vi "CalcLift.vi"(5 "Teleop Local Data In":T1 {"Vision"."Theta_Y" format="%.1f"; "Vision"."Theta_X" format="%.1f"; "Potentio" format="%.1f"; "Drive_Enc_R" format="%.1f"; "Drive_Enc_L" format="%.1f"; "Gyro_Angle" format="%.1f"; "Encoder_Lift" format="%.1f"; "Motor_Lift" format="%.3f"; "Motor_Intake" format="%.3f"; "Drive_Twist" format="%.3f"; "Drive_Forward" format="%.3f"}, 9 "error in":errorcluster) -> (6 "Teleop Local Data Out":T1 {"Vision"."Theta_Y" format="%.1f"; "Vision"."Theta_X" format="%.1f"; "Potentio" format="%.1f"; "Drive_Enc_R" format="%.1f"; "Drive_Enc_L" format="%.1f"; "Gyro_Angle" format="%.1f"; "Encoder_Lift" format="%.1f"; "Motor_Lift" format="%.3f"; "Motor_Intake" format="%.3f"; "Drive_Twist" format="%.3f"; "Drive_Forward" format="%.3f"}, 10 "error out":errorcluster)   [LabVIEW 2018]
uses:
  Typedefs/typedef_cluster_TeleOp_Local_Data.ctl
  Typedefs/typedef_cluster_Joystick.ctl
  Typedefs/typedef_cluster_Vision.ctl
  Typedefs/typedef_enum_refnums.ctl
  <vilib>/Rock Robotics/WPI/ThirdParty/Phoenix-LabVIEW/Motor Controller/Get/CTRE_Phoenix_MotorController_GetQuadratureData.vi
  <vilib>/Rock Robotics/WPI/ThirdParty/Phoenix-LabVIEW/Motor Controller/Get/CTRE_Phoenix_MotorController_GetLimitSwitchStates.vi
panel:
  in  "K Down":dbl=8.0
  in  "K":dbl=5.0
  in  "lower limit":dbl
  in  "upper limit":dbl=2700.0
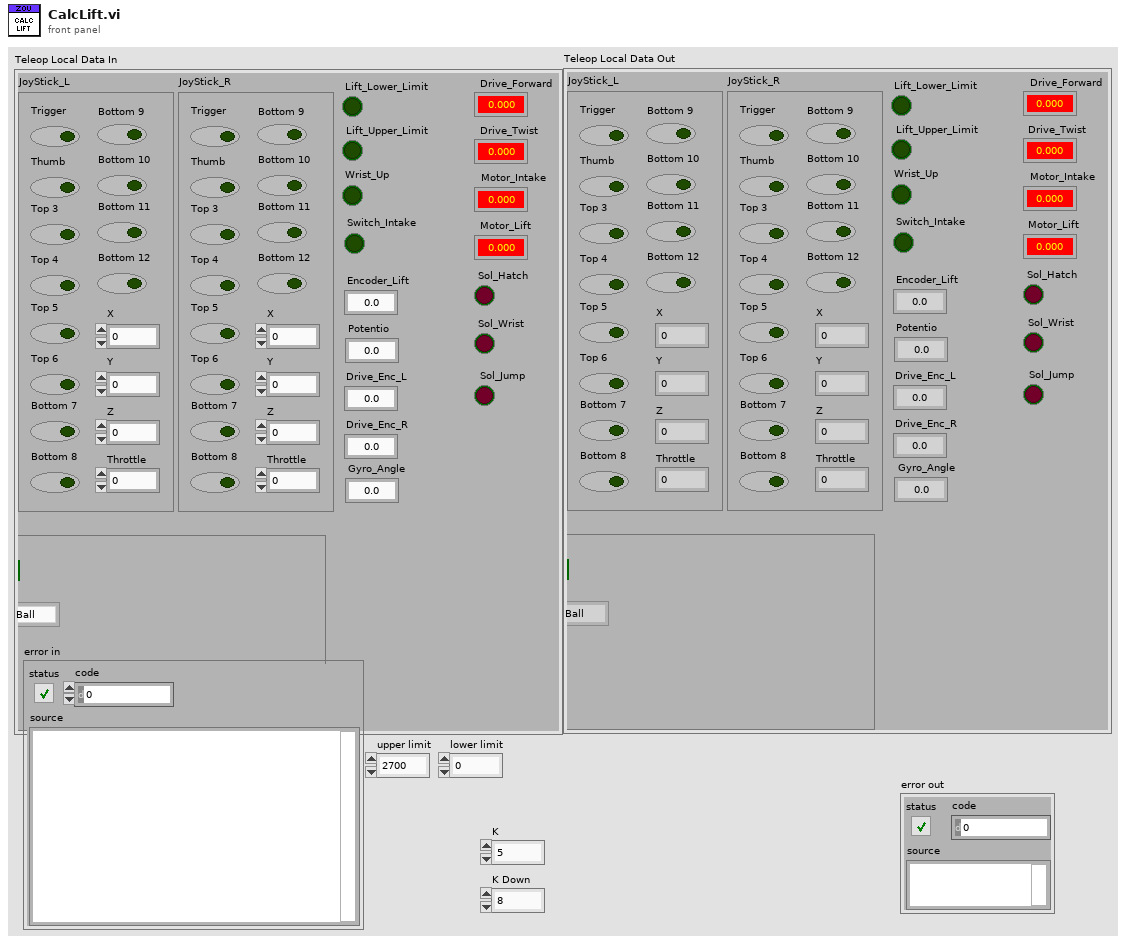
[diagram p1: front panel]
types:
  T1 = typedef "typedef_cluster_TeleOp_Local_Data.ctl" = cluster{"Lift_Lower_Limit":bool, "Wrist_Up":bool, "Switch_Intake":bool, "Encoder_Lift":dbl, "Sol_Wrist":bool, "Motor_Intake":dbl, "Motor_Lift":dbl, "Drive_Forward":dbl, "Drive_Twist":dbl, "Sol_Hatch":bool, "Gyro_Angle":dbl, "Drive_Enc_L":dbl, "Drive_Enc_R":dbl, "JoyStick_L":T2, "JoyStick_R":T2, "Potentio":dbl, "Vision":T3, "Lift_Upper_Limit":bool, "Sol_Jump":bool}
  T2 = typedef "typedef_cluster_Joystick.ctl" = cluster{"X":dbl, "Y":dbl, "Z":dbl, "Throttle":dbl, "Trigger":bool, "Thumb":bool, "Top 3":bool, "Top 4":bool, "Top 5":bool, "Top 6":bool, "Bottom 7":bool, "Bottom 8":bool, "Bottom 9":bool, "Bottom 10":bool, "Bottom 11":bool, "Bottom 12":bool}
  T3 = typedef "typedef_cluster_Vision.ctl" = cluster{"Theta_X":dbl, "Theta_Y":dbl, "Has_Target":bool, "Seek_Ball":bool, "Pipeline":enum16{"Ball", "Dual_Target", "Single_Target"}}
  T4 = typedef "typedef_enum_refnums.ctl" = enum16{"Joy_L", "Joy_R", "Drive_Motors", "Intake_Motor", "Wrist_Solenoid", "Hatch_Solenoid", "Compressor", "Lift_Motor", "Lift_Motor_2", "Gyro", "Drive_Enc_L", "Drive_Enc_R", "Lift_Lower_Limit", "Lift_Upper_Limit", "Ball_Switch", "Jump_Solenoid"}
  T5 = typedef "WPI_MotorControlDeviceRef.ctl" = cluster{"DeviceStatus":errorcluster, "Type":T6, "PWM":cluster{"PWM Channel":T7, "DeadBand":T8}, "CAN":cluster{"Device Number":u8, "SetOutput VI Ref":variant, "GetOutput VI Ref":variant, "Enable VI Ref":variant, "Disable VI Ref":variant, "Data":variant}, "Invert":bool, "DIO PWM":cluster{"PWM \"Enable\" Channel":T7, "DIOChannel":T9, "PWM Rate":dbl}}
  T6 = typedef "WPI_MotorControlType.ctl" = enum16{"PWM", "CAN", "DIO PWM"}
  T7 = typedef "FPGA_DIOPWMChannel.ctl" = enum8{"PWM 0", "PWM 1", "PWM 2", "PWM 3", "PWM 4", "PWM 5", "PWM 6", "PWM 7", "PWM 8", "PWM 9", "PWM MXP 0", "PWM MXP 1", "PWM MXP 2", "PWM MXP 3", "PWM MXP 4", "PWM MXP 5", "PWM MXP 6", "PWM MXP 7", "PWM MXP 8", "PWM MXP 9", "Invalid"}
  T8 = typedef "WPI_PWMDeadband.ctl" = cluster{"Name":string, "maxPositivePwm":i32, "minPositivePwm":i32, "centerPwm":i32, "maxNegativePwm":i32, "minNegativePwm":i32, "angularRange":u16}
  T9 = typedef "FPGA_DIOChannel.ctl" = enum8{"DIO 0", "DIO 1", "DIO 2", "DIO 3", "DIO 4", "DIO 5", "DIO 6", "DIO 7", "DIO 8", "DIO 9", "DIO MXP 0", "DIO MXP 1", "DIO MXP 2", "DIO MXP 3", "DIO MXP 4", "DIO MXP 5", "DIO MXP 6", "DIO MXP 7", "DIO MXP 8", "DIO MXP 9", "DIO MXP 10", "DIO MXP 11", "DIO MXP 12", "DIO MXP 13", "DIO MXP 14", "DIO MXP 15", "SPI Port CS1", "SPI Port CS2", "SPI Port CS3", "SPI Port MISO", "SPI Port MOSI", "Invalid"}
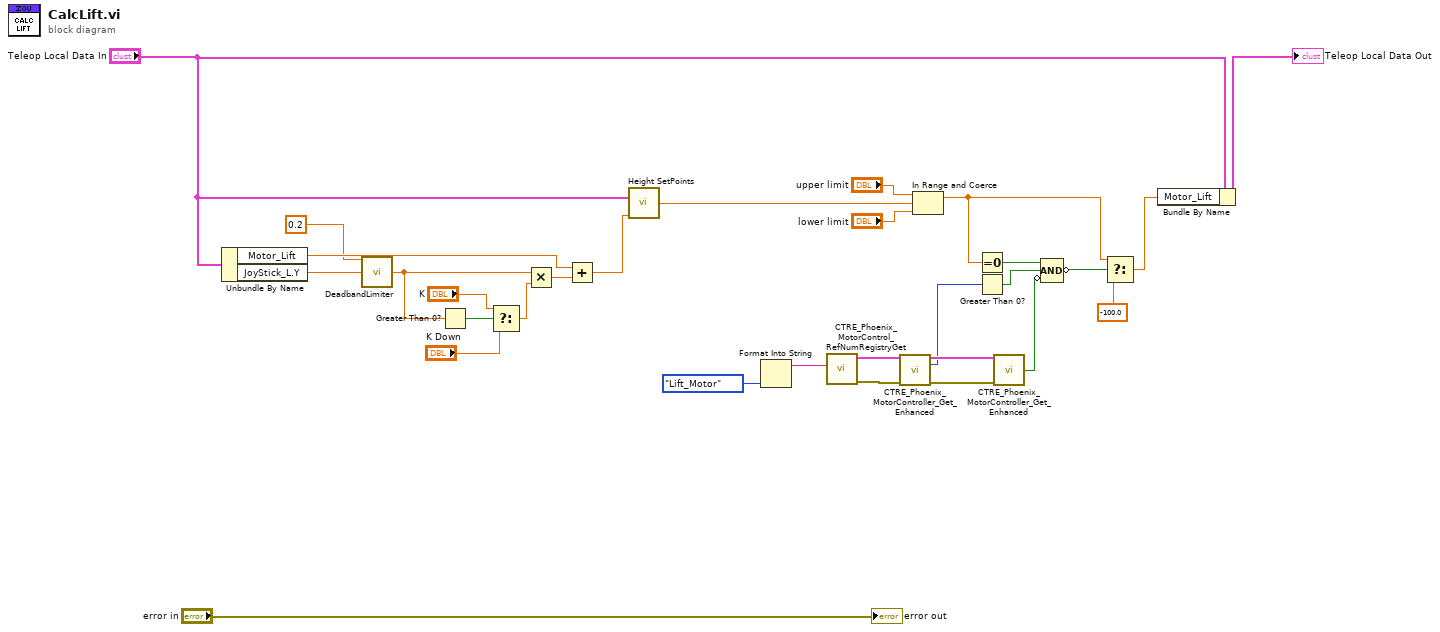
[diagram p0: block diagram]
diagram:
  n1 = Unbundle By Name("Teleop Local Data In") -> ("Motor_Lift"=w19:dbl, "JoyStick_L.Y"=w23:dbl)
  n2 = call "DeadbandLimiter.vi"("Deadband Percentage"=0.2, "Input"=w23) -> ("Deadband Output"=w22:dbl)  [unwired: 13 in]
  n3 = Greater Than 0?(x=w22) -> (x > 0?=w26:bool)
  n4 = Select(t="K", s=w26, f="K Down") -> (s? t:f=w21:dbl)
  n5 = Multiply(x=w22, y=w21) -> (x*y=w20:dbl)
  n6 = Add(x=w19, y=w20) -> (x+y=w5:dbl)
  n7 = call "Height SetPoints.vi"("Teleop Local Data In"="Teleop Local Data In", "Manual Drive Input"=w5) -> ("Set Point out"=w6:dbl)  [unwired: 13 in]
  n8 = Format Into String(typedef_enum_refnums."Lift_Motor" ("Enum")) -> (resulting string=w18:string)  [unwired: 3 in, 1 out]
  n9 = call <vilib>:"CTRE_Phoenix_MotorControl_RefNumRegistryGet.vi"("refnum name"=w18) -> ("error out"=w1:errorcluster, "PhoenixMotorControlDevRef"=w2:T5)  [unwired: 9 in]
  n10 = call-poly <vilib>:"CTRE_Phoenix_MotorController_Get_Enhanced.vi"("PhoenixMotorControlDevRef"=w2, "error in"=w1) -> ("PhoenixMotorControlDevRef"=w16:T5, "Quadrature Position"=w13:i32, "error out"=w15:errorcluster)  [unwired: 10 in, 1 out]
  n11 = In Range and Coerce(upper limit="upper limit", x=w6, lower limit="lower limit") -> (coerced(x)=w10:dbl)  [unwired: 1 out]
  n12 = Equal To 0?(x=w10) -> (x = 0?=w14:bool)
  n13 = Greater Than 0?(x=w13) -> (x > 0?=w12:bool)
  n14 = call-poly <vilib>:"CTRE_Phoenix_MotorController_Get_Enhanced.vi"("PhoenixMotorControlDevRef"=w16, "error in"=w15) -> ("Reverse Limit Closed?"=w7:bool)  [unwired: 10 in, 3 out]
  n15 = Compound Arithmetic op=AND(w14, w12, invert w7) -> (invert w11:bool)
  n16 = Select(t=w10, s=w11, f=-100.0) -> (s? t:f=w9:dbl)
  n17 = Bundle By Name(cluster="Teleop Local Data In", "Motor_Lift"=w9) -> (→"Teleop Local Data Out":T1)
  "error out" <- "error in"
